vi "Inheritance Main.vi"() -> ()   [LabVIEW 2009, in "HB_Inherance_Example.lvlib"]
doc: "This VI is used to demonstrate inheritance."
uses:
  HB_Inherance_Example.lvlib
  HB_TwoButtonDiolog/HB_TwoButtonDiolog.lvclass
  HB_OneButtonDialog/HB_OneButtonDialog.lvclass
  HB_Dialog/HB_Dialog.lvclass
  lib.lib/HGF_LVC/HGF_Auxiliary/HGF_Auxiliary.lvlib
panel:
  in  "NofButtons":i16=1 min=0 step=1
  out "canceled":bool
  out "Button Index":i16
  in  "OO?":bool
  in  "F button name (\"Cancel\")":string="Cancel"
  in  "T button name (\"OK\")":string="OK"
  in  "Message":string
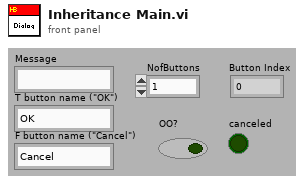
[diagram p1: front panel]
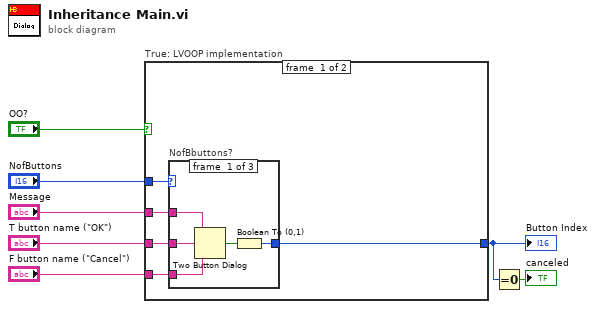
[diagram p0: block diagram]
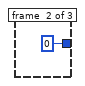
[diagram p2: hidden frame]
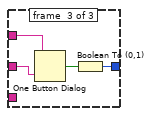
[diagram p3: hidden frame]
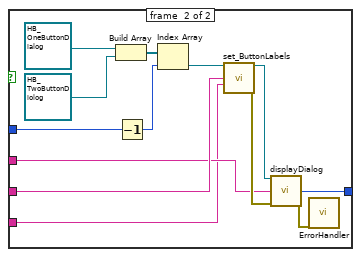
[diagram p4: hidden frame]
diagram:
  n1 = case "True: LVOOP implementation" shown="True" "OO?" {
    tunnel: "NofButtons" -> [w12 w28]
    tunnel: "Message" -> [w11 w25]
    tunnel: "T button name (\"OK\")" -> [w10 w26]
    tunnel: "F button name (\"Cancel\")" -> [w9 w24]
    tunnel: [w8 w34] -> w2
    frame #0 {
      n2 = case "NofBbuttons?" shown="2" w12 {
        tunnel: w11 -> [w17 _ w21]
        tunnel: w10 -> [w16 _ w20]
        tunnel: w9 -> [w15 _ _]
        tunnel: [w13 i16 0 w19] -> w8
        frame #0 {
          n3 = Two Button Dialog(message=w17, 1:w15, 2:w16) -> (T button?=w14:bool)
          n4 = Boolean To (0,1)(Boolean=w14) -> (0, 1=w13:i16)
        }
        frame #1 {
        }
        frame #2 {
          n5 = One Button Dialog(message=w21, button name ("OK")=w20) -> (true=w22:bool)
          n6 = Boolean To (0,1)(Boolean=w22) -> (0, 1=w19:i16)
        }
      }
    }
    frame #1 {
      n7 = Build Array(refnum<class "HB_OneButtonDialog.lvclass"> refnum ("HB_OneButtonDialog.lvclass"), refnum<class "HB_TwoButtonDiolog.lvclass"> refnum ("HB_TwoButtonDiolog.lvclass")) -> (w33:refnum<class "HB_Dialog.lvclass">[])
      n8 = Decrement(x=w28) -> (x-1=w27:i16)
      n9 = Index Array(array=w33, index=w27) -> (element=w23:refnum<class "HB_Dialog.lvclass">)
      n10 = call "set_ButtonLabels.vi"("HB_Dialog in"=w23, "T button name (\"OK\")"=w26, "F button name (\"Cancel\")"=w24) -> ("HB_Dialog out"=w32:refnum<class "HB_Dialog.lvclass">, "error out"=w31:errorcluster)  [unwired: 11 in]
      n11 = call-dynamic "displayDialog.vi"("HB_Dialog in"=w32, "Message"=w25, "error in (no error)"=w31) -> ("Button Index"=w34:i16, "error out"=w35:errorcluster)  [unwired: 10 in, 1 out]
      n12 = call "ErrorHandler.vi"("error in (no error)"=w35) -> ()  [unwired: 13 in, 6 out]
    }
  }
  "Button Index" <- w2
  n13 = Equal To 0?(x=w2) -> (x = 0?=→"canceled":bool)
